vi "Inverse Dynamics.vi"(10 "Jacobian Matrix":T1, 11 "F desired Matrix":T1) -> (2 "Reference Tension":dbl[](array[numeric]))   [LabVIEW 2021]
uses:
  <vilib>/Analysis/Matrix/Datatypes/RealMatrix.ctl
  <vilib>/Analysis/_algsub.llb/Real PseudoInverse Matrix.vi
  <vilib>/Analysis/baseanly.llb/Real A x B.vi
  <vilib>/Analysis/Matrix/Numeric/Conversions/Matrix To Array - RM.vi
  <vilib>/Analysis/NI_AALPro.lvlib
  <vilib>/Analysis/NI_AALBase.lvlib
  <vilib>/Analysis/Matrix/NI_Matrix.lvlib
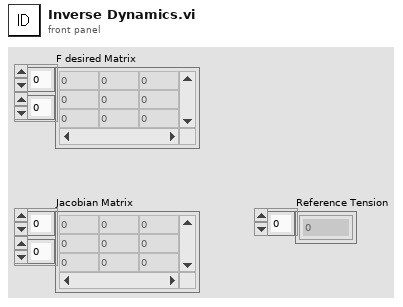
[diagram p1: front panel]
types:
  T1 = typedef "NI_Matrix.lvlib/RealMatrix.ctl" = dbl[][]
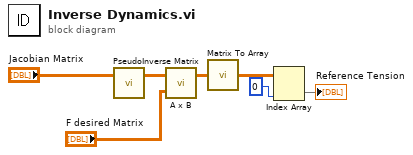
[diagram p0: block diagram]
diagram:
  n1 = call-poly <vilib>:"PseudoInverse Matrix.vi"("Input Matrix"="Jacobian Matrix") -> ("PseudoInverse Matrix"=w1:T1)  [unwired: 1 in, 1 out]
  n2 = call-poly <vilib>:"A x B.vi"("B"="F desired Matrix", "A"=w1) -> ("A x B"=w2:T1)  [unwired: 1 out]
  n3 = call-poly <vilib>:"Matrix To Array.vi"("Real Matrix"=w2) -> ("Real 2D Array"=w3:dbl[][])
  n4 = Index Array(array=w3, index (col)=0 ("index")) -> (element=→"Reference Tension":dbl[])  [unwired: 1 in]
